vi "Front Camera Circle detect.vi"() -> ()   [LabVIEW 2014]
uses:
  <vilib>/vision/Shape Detection.llb/ShapeDetectionMatchOptions.ctl
  <vilib>/vision/Pattern Matching.llb/IMAQ Match Range Setting.ctl
  <vilib>/vision/Pattern Matching.llb/IMAQ Curve Parameters.ctl
  Others (.ctl)/Control cluster.ctl
  Global.vi
  <vilib>/vision/NI_Vision_Development_Module.lvlib
panel:
  out "Score":dbl
  out "Number of Matches Returned":i32
  in  "Curve Parameters":T1={"Extraction Mode"=0, "Edge Threshold"=150, "Edge Filter Size"=1, "Min Length"=25, "Row Search Step Size"=15, "Col Search Step Size"=15, "Max Endpoint Gap"=10, "Closed"=TRUE, "Subpixel"=FALSE} {"Extraction Mode" items=["Normal", "Uniform Regions"]; "Edge Filter Size" items=["Fine", "Normal", "Contour Tracing"]; "Max Endpoint Gap" min=0; "Col Search Step Size" min=1 max=255 step=1; "Row Search Step Size" min=1 max=255 step=1; "Min Length" min=0; "Edge Threshold" min=1 max=350 step=1}
  out "error out":errorcluster
  in  "Minimum match score":dbl=900.0
  in  "Match Options":T2={"Rotation"=FALSE, "Scale"=FALSE, "Occlusion"=TRUE, "Range Settings"=[{"Match Constraints"=0, "Min"=0.0, "Max"=0.0}, {"Match Constraints"=1, "Min"=0.0, "Max"=0.0}, {"Match Constraints"=2, "Min"=0.0, "Max"=25.0}]} {"Range Settings"."Max" format="%.2f"; "Range Settings"."Min" format="%.2f"; "Range Settings"."Match Constraints" items=["Rotation Angle (degrees)", "Scale Factor (%)", "Occlusion (%)"]}
  in  "Circle Descriptor":cluster{"Min Radius":dbl, "Max Radius":dbl}={"Min Radius"=20.0, "Max Radius"=400.0}
  out "Image":T4(plugin-control)
  in  "stop video":bool
  in  "milliseconds to wait":u32
  out "Read Video":errorcluster
  out "x-y":u32=19
  # "Range"
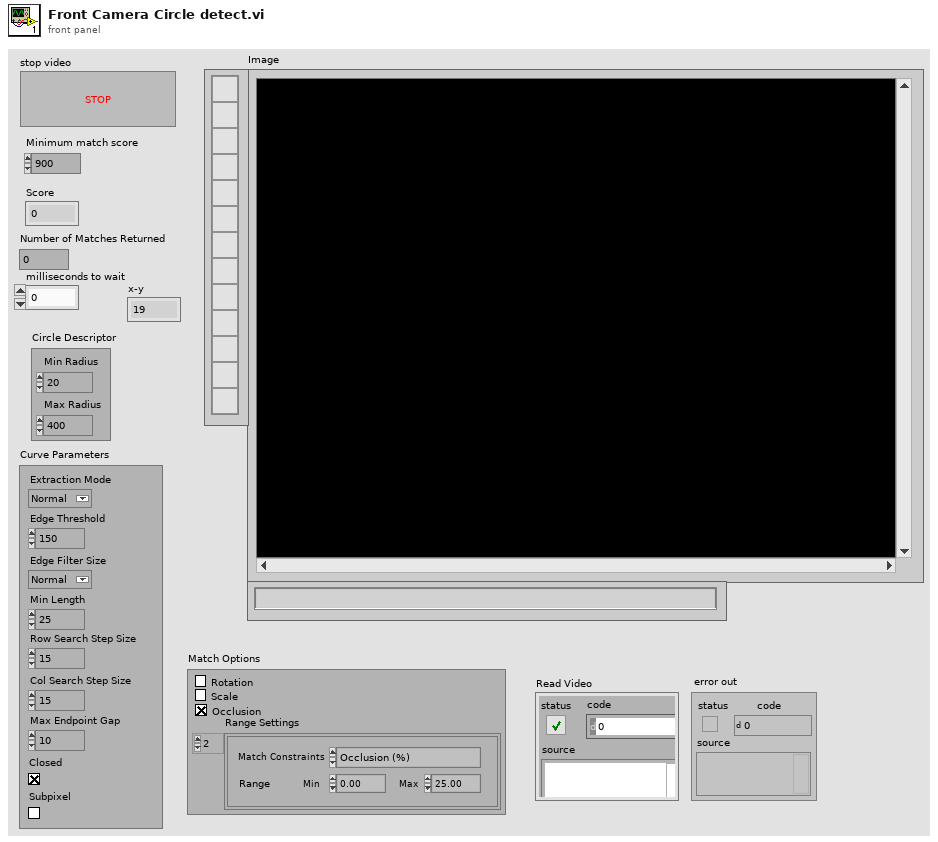
[diagram p1: front panel]
types:
  T1 = typedef "IMAQ Curve Parameters.ctl" = cluster{"Extraction Mode":u32, "Edge Threshold":i32, "Edge Filter Size":u32, "Min Length":i32, "Row Search Step Size":i32, "Col Search Step Size":i32, "Max Endpoint Gap":i32, "Closed":bool, "Subpixel":bool}
  T2 = typedef "ShapeDetectionMatchOptions.ctl" = cluster{"Rotation":bool, "Scale":bool, "Occlusion":bool, "Range Settings":T3[]}
  T3 = typedef "IMAQ Match Range Setting.ctl" = cluster{"Match Constraints":u32, "Min":dbl, "Max":dbl}
  T4 = typedef "IMAQ Image.ctl" = refnum<image>
  T5 = typedef "Control cluster.ctl" = cluster{"Roll":sgl, "Pitch":sgl, "Vertical Speed":sgl, "Yaw Speed":sgl}
  T6 = typedef "Image Type" = u32
  T7 = cluster{"Position":cluster{"X":sgl, "Y":sgl}, "Radius":dbl, "Score":dbl}[]
  T8 = cluster{"Position":cluster{"X":sgl, "Y":sgl}, "Radius":dbl, "Score":dbl}
  T9 = cluster{"Left":i32, "Top":i32, "Right":i32, "Bottom":i32}
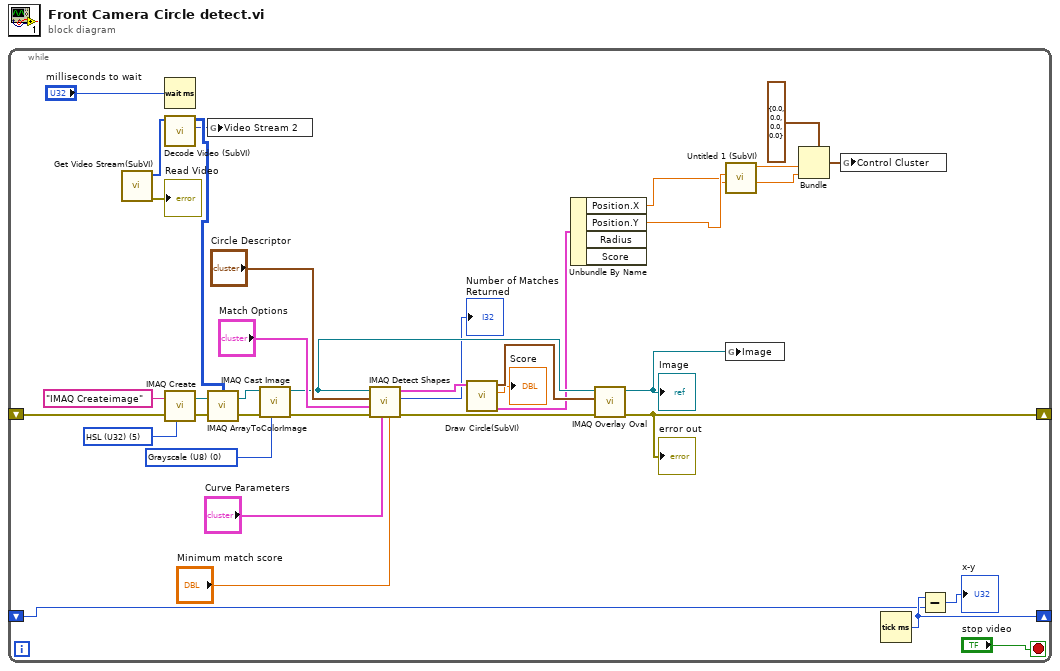
[diagram p0: block diagram]
diagram:
  n1 = while {
    shift-right: [w28] -> _
    shift-left: _ -> [w27]
    shift-right: [w13] -> _
    shift-left: _ -> [w24]
    stop <- "stop video" stop-if-true
    w21 = T6 0 items=["Grayscale (U8)", "Grayscale (I16)", "Grayscale (SGL)", "Complex (CSG)", "RGB (U32)", "HSL (U32)", "RGB (U64)", "Grayscale (U16)"] ("Image Type")
    w34 = T6 5 items=["Grayscale (U8)", "Grayscale (I16)", "Grayscale (SGL)", "Complex (CSG)", "RGB (U32)", "HSL (U32)", "RGB (U64)", "Grayscale (U16)"] ("Image Type")
    n2 = call "Get Video Stream(SubVI).vi"() -> ("error out"=→"Read Video":errorcluster, "ImgData"=w35:u8[])  [unwired: 10 in]
    n3 = Wait (ms)(milliseconds to wait="milliseconds to wait") -> ()  [unwired: 1 out]
    n4 = call "Decode Video (SubVI).vi"("ImgData"=w35) -> ("new picture"=w25:picture, "Array"=w31:u32[][])  [unwired: 9 in]
    n5 = call "IMAQ Create"("Image Name"="IMAQ Createimage", "Image Type"=w34, "error in (no error)"=w24) -> ("New Image"=w30:T4, "error out"=w29:errorcluster)  [unwired: 2 in]
    n6 = global write "Global.vi" "Video Stream 2"(w25) -> ()
    n7 = call "IMAQ ArrayToColorImage"("Image Pixels (U32)"=w31, "Image"=w30, "error in (no error)"=w29) -> ("Image Out"=w22:T4, "error out"=w23:errorcluster)  [unwired: 2 in]
    n8 = call "IMAQ Cast Image"("Image Type"=w21, "error in (no error)"=w23, "Image Src"=w22) -> ("error out"=w18:errorcluster, "Image Dst Out"=w16:T4)  [unwired: 7 in]
    n9 = call-poly "IMAQ Detect Shapes"("Minimum match score"="Minimum match score", "Curve Parameters"="Curve Parameters", "error in (no error)"=w18, "Match Options"="Match Options", "Circle Descriptor"="Circle Descriptor", "Image"=w16) -> ("error out"=w15:errorcluster, "Number of Matches Returned"=→"Number of Matches Returned":i32, "Circles"=w11:T7)  [unwired: 3 in]
    n10 = call "Draw Circle(SubVI).vi"("Circles"=w11) -> ("element"=w8:T8, "Score"=→"Score":dbl, "Bounding Rectangle out"=w14:T9)  [unwired: 8 in]
    n11 = Unbundle By Name(w8) -> ("Position.X"=w1:sgl, "Position.Y"=w2:sgl)  [unwired: 2 out]
    n12 = call "IMAQ Overlay Oval"("error in (no error)"=w15, "Bounding Rectangle"=w14, "Image"=w16) -> ("error out"=w13:errorcluster, "Image Out"=w3:T4)  [unwired: 7 in]
    "Image" <- w3
    "error out" <- w13
    n13 = call "Untitled 1 (SubVI).vi"("X"=w1, "Y"=w2) -> ("Roll"=w4:dbl, "Pitch"=w5:dbl)  [unwired: 7 in, 1 out]
    n14 = global write "Global.vi" "Image"(w3) -> ()
    n15 = Bundle(cluster=T5 {"Roll"=0.0, "Pitch"=0.0, "Vertical Speed"=0.0, "Yaw Speed"=0.0} ("Control Cluster"), "Vertical Speed"=w5, "Yaw Speed"=w4) -> (w7:T5)  [unwired: 2 in]
    n16 = global write "Global.vi" "Control Cluster"(w7) -> ()
    n17 = Tick Count (ms)() -> (millisecond timer value=w28:u32)
    n18 = Subtract(x=w28, y=w27) -> (x-y=→"x-y":u32)
  }
